vi "Destroy Request Events.vi"(8 "error in (no error)":errorcluster) -> (0 "error out":errorcluster)   [LabVIEW 2021, in "Actuator Module.lvlib"]
doc: "Destroy the requests user events, even if there is an incoming error.\n\n<b>NOTE</b>: The contents of this VI are automatically generated and modified by the <b>Tools > Delacor > User Event</b> utilities. Consider using those utilities instead of making your own modifications to this VI.\n_______\nCreated using Delacor User Event Scripter 1.0.0.6."
uses:
  Actuator Module.lvlib
panel:
  # "NOTE: The contents of this VI are automatically generated and modified by the Tools > Delacor > User Event utilities. Consider using those utilities instead of making your own modifications to this VI."
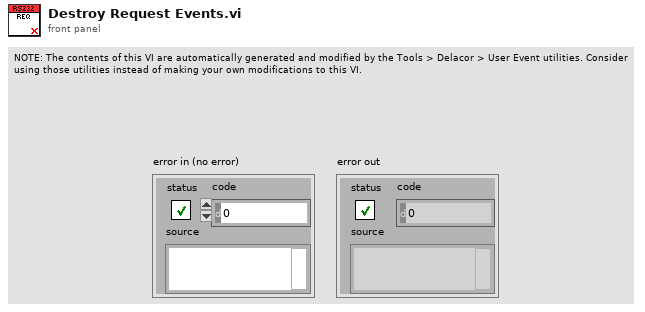
[diagram p1: front panel]
types:
  T1 = typedef "Actuator Module.lvlib/Request Events--cluster.ctl" = cluster{"Stop":refnum<user-event>, "Set Actuator":refnum<user-event>}
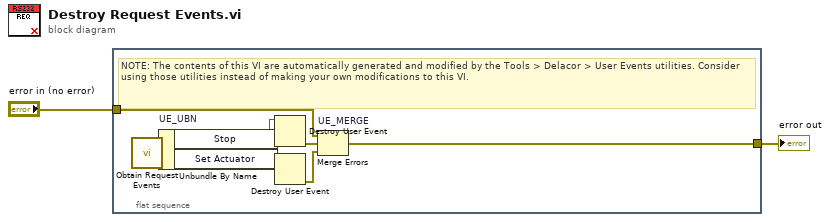
[diagram p0: block diagram]
diagram:
  n1 = flat-sequence {
    tunnel: [w9] -> w2
    tunnel: "error in (no error)" -> [w5]
    frame #0 {
      # "NOTE: The contents of this VI are automatically generated and modified by the Tools > Delacor > User Events utilities. Consider using those utilities instead of making your own modifications to this VI."
      n2 = call "Obtain Request Events.vi"() -> ("Actuator Module Request Events"=w8:T1)  [unwired: 10 in, 1 out]
      n3 = Unbundle By Name "UE_UBN"(w8) -> ("Stop"=w7:refnum<user-event>, "Set Actuator"=w3:refnum<user-event>)
      n4 = Destroy User Event(user event=w7) -> (error out=w6:errorcluster)  [unwired: 1 in]
      n5 = Destroy User Event(user event=w3) -> (error out=w4:errorcluster)  [unwired: 1 in]
      n6 = Merge Errors "UE_MERGE"(w5, w6, w4) -> (w9:errorcluster)
    }
  }
  "error out" <- w2
